vi "AddSystemDataConfiguration.vi"(6 "argument":i32, 8 "error in (no error)":errorcluster, 9 "system data signal":u32(ring)=74 items=["DataCollectionSampleIndex"=161, "DataCollectionSampleTime"=149, "DataCollectionStatus"=255, "DriveModbusMasterInputBits"=354, "DriveModbusMasterInputWords"=352, "DriveModbusMasterOutputBits"=355, "DriveModbusMasterOutputStatusBits"=356, "DriveModbusMasterOutputStatusWords"=357, "DriveModbusMasterOutputWords"=353, "EstimatedProcessorUsage"=236, "FieldbusActiveConnections"=287, "FieldbusConnected"=284, "FieldbusErrorCode"=285, "FieldbusErrorLocation"=286, "FieldbusInactiveConnections"=288, "FieldbusInputs"=340, "FieldbusOutputs"=341, "GlobalVariable"=74, "LibraryCommand"=148, "ModbusMasterInputBits"=344, "ModbusMasterInputWords"=342, "ModbusMasterOutputBits"=345, "ModbusMasterOutputStatusBits"=346, "ModbusMasterOutputStatusWords"=347, "ModbusMasterOutputWords"=343, "ModbusSlaveInputBits"=350, "ModbusSlaveInputWords"=348, "ModbusSlaveOutputBits"=351, "ModbusSlaveOutputWords"=349, "PCModbusMasterConnected"=170, "PCModbusMasterErrorCode"=174, "PCModbusMasterErrorLocation"=176, "PCModbusSlaveConnected"=171, "PCModbusSlaveErrorCode"=175, "PCModbusSlaveErrorLocation"=177, "PLCBool"=211, "PLCByte"=212, "PLCDint"=217, "PLCDword"=214, "PLCInt"=216, "PLCLreal"=222, "PLCReal"=221, "PLCSint"=215, "PLCUdint"=220, "PLCUint"=219, "PLCUsint"=218, "PLCWord"=213, "SafeZoneActiveMask"=321, "SafeZoneViolationMask"=289, "ScopetrigID"=209, "SignalLogState"=270, "StopWatchTimer"=197, "SystemParameter"=379, "Timer"=56, "TimerPerformance"=57, "VirtualBinaryInput"=51, "VirtualBinaryOutput"=52, "VirtualRegisterInput"=53, "VirtualRegisterOutput"=54, "ZYGOPosition1"=164, "ZYGOPosition2"=165, "ZYGOPosition3"=166, "ZYGOPosition4"=167], 11 "controller in":refnum<k24>) -> (0 "error out":errorcluster, 3 "controller out":refnum<k24>)   [LabVIEW 2016, in "Aerotech VIs.lvlib"]
uses:
  Aerotech VIs.lvlib
  C:/Program Files (x86)/Aerotech/A3200/LabVIEW/2010/Bin/Aerotech.A3200.dll
  C:/Program Files (x86)/Aerotech/A3200/LabVIEW/2010/Bin/Aerotech.A3200.LabVIEW.dll
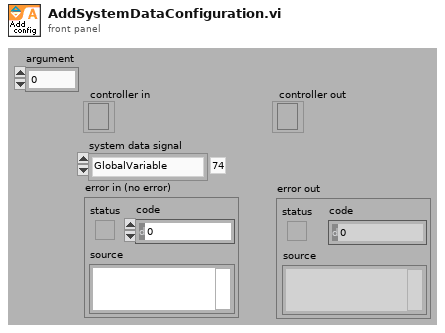
[diagram p1: front panel]
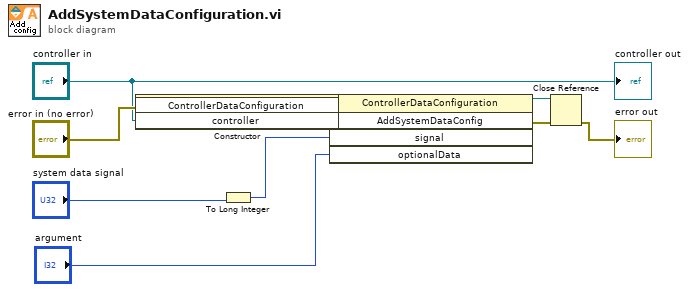
[diagram p0: block diagram]
diagram:
  n1 = constructor class="ControllerDataConfiguration"(error in="error in (no error)", "controller"="controller in") -> (reference out=w9:refnum<k24>, error out=w8:errorcluster)  [unwired: 2 in, 2 out]
  n2 = To Long Integer(number="system data signal") -> (32bit integer=w3:i32)
  n3 = invoke class="ControllerDataConfiguration" method="AddSystemDataConfig"(reference=w9, error in=w8, "signal"=w3, "optionalData"="argument") -> (reference out=w6:refnum<k24>, error out=w5:errorcluster)  [unwired: 1 in, 3 out]
  n4 = Close Reference(reference=w6, error in (no error)=w5) -> (error out=→"error out":errorcluster)
  "controller out" <- "controller in"
